vi "log analysis_gps.vi"() -> ()   [LabVIEW 2018] (continued)
2 27.900000 0 0\trobot status\t233.917361\t102.956881\t8.394900\t0.257932\t-0.250093\t-19.886143\t0.214000\t0.155000\n\t\n15:20:07.4\tlog_raw\tgps_raw\t\tsystem status\tnormal 2 27.900000 0 0\trobot status\t234.044213\t102.902455\t8.392800\t0.335822\t-0.062478\t-19.109713\t0.317000\t-0.011000\n\t\n15:20:07.9\tlog_raw\tgps_raw\t\tsystem status\tnormal 2 27.900000 0 0\trobot status\t234.173574\t102.852025\t8.391200\t0.185875\t0.011121\t-18.240384\t0.261000\t0.072000\n\t\n15:20:08.4\tlog_raw\tgps_raw\t\tsystem status\tnormal 2 27.900000 0 0\trobot status\t234.306855\t102.799992\t8.389600\t0.221268\t0.001420\t-17.502201\t0.351000\t-0.068000\n\t\n15:20:08.9\tlog_raw\tgps_raw\t#INSPVAXA,USB3,0,49.0,FINESTEERING,2107,282026.900,02000000,471d,15824;INS_ALIGNMENT_COMPLETE,INS_RTKFIXED,37.37105597447,126.72348196925,8.3886,22.3000,-0.1101,0.2823,-0.0032,0.311492548,-0.004113518,106.939400218,0.4050,0.2960,0.5269,0.1087,0.0927,0.0760,0.1504,0.1513,4.9517,0f000001,0*e3da5464\n\tsystem status\tnormal 2 27.900000 0 0\trobot status\t234.454891\t102.743810\t8.388600\t0.311493\t-0.004114\t-16.939400\t0.243000\t0.103000\n\t\n15:20:09.4\tlog_raw\tgps_raw\t\tsystem status\tnormal 2 27.900000 0 0\trobot status\t234.572623\t102.698923\t8.387800\t0.503029\t-0.025580\t-16.641655\t0.366000\t-0.093000\n\t\n15:20:09.9\tlog_raw\tgps_raw\t\tsystem status\tnormal 2 28.000000 0 0\trobot status\t234.705268\t102.650315\t8.386900\t0.470119\t-0.136101\t-16.414605\t0.222000\t0.114000\n\t\n15:20:10.4\tlog_raw\tgps_raw\t\tsystem status\tnormal 2 28.000000 0 0\trobot status\t234.841052\t102.602660\t8.385400\t0.352834\t-0.219751\t-16.257896\t0.249000\t0.066000\n\t\n15:20:10.9\tlog_raw\tgps_raw\t#INSPVAXA,USB3,0,48.5,FINESTEERING,2107,282028.900,02000000,471d,15824;INS_ALIGNMENT_COMPLETE,INS_RTKFIXED,37.37105423586,126.72348799189,8.3853,22.3000,-0.0954,0.2609,0.0063,0.345591384,-0.136100185,106.270510244,0.4039,0.2954,0.5254,0.1083,0.0924,0.0759,0.1502,0.1513,4.9544,0f000001,0*0554cafd\n\tsystem status\tnormal 2 28.100000 0 0\trobot status\t234.988367\t102.550836\t8.385300\t0.345591\t-0.136100\t-16.270510\t0.353000\t-0.085000\n\t\n15:20:11.4\tlog_raw\tgps_raw\t#INSPVAXA,USB3,0,51.5,FINESTEERING,2107,282029.400,02000000,471d,15824;INS_ALIGNMENT_COMPLETE,INS_RTKFIXED,37.37105381452,126.72348943964,8.3855,22.3000,-0.0956,0.2580,0.0057,0.437004372,-0.047146220,106.316911709,0.4029,0.2951,0.5243,0.1082,0.0924,0.0758,0.1501,0.1513,4.9556,0f000001,0*8a2f1e39\n\tsystem status\tnormal 2 28.100000 0 0\trobot status\t235.116606\t102.504071\t8.385500\t0.437004\t-0.047146\t-16.316912\t0.290000\t-0.013000\n\t\n15:20:11.9\tlog_raw\tgps_raw\t\tsystem status\tnormal 2 28.100000 0 0\trobot status\t235.235324\t102.460737\t8.385200\t0.512593\t-0.025982\t-16.425226\t0.294000\t-0.033000\n\t\n15:20:12.4\tlog_raw\tgps_raw\t\tsystem status\tnormal 2 28.100000 0 0\trobot status\t235.364702\t102.414096\t8.385200\t0.428006\t0.220406\t-16.561656\t0.296000\t-0.023000\n\t\n15:20:12.9\tlog_raw\tgps_raw\t\tsystem status\tnormal 2 28.100000 0 0\trobot status\t235.492637\t102.367047\t8.386000\t0.390693\t0.448694\t-16.706600\t0.298000\t-0.026000\n\t\n15:20:13.4\tlog_raw\tgps_raw\t\tsystem status\tnormal 2 28.100000 0 0\trobot status\t235.625886\t102.316793\t8.387700\t0.367788\t0.548182\t-16.923819\t0.298000\t-0.028000\n\t\n15:20:13.9\tlog_raw\tgps_raw\t\tsystem status\tnormal 2 28.100000 0 0\trobot status\t235.772529\t102.261880\t8.389500\t0.368907\t0.593009\t-17.130750\t0.304000\t-0.029000\n\t\n15:20:14.4\tlog_raw\tgps_raw\t#INSPVAXA,USB3,0,49.5,FINESTEERING,2107,282032.400,02000000,471d,15824;INS_ALIGNMENT_COMPLETE,INS_RTKFIXED,37.37105111138,126.72349854734,8.3925,22.3000,-0.1007,0.2882,0.0025,0.307227666,0.473154463,107.541908960,0.4011,0.2941,0.5198,0.1079,0.0924,0.0756,0.1501,0.1513,4.9577,0f000001,0*dbe53f25\n\tsystem status\tnormal 2 28.100000 0 0\trobot status\t235.923351\t102.204041\t8.392500\t0.307228\t0.473154\t-17.541909\t0.297000\t-0.033000\n\t\n15:20:14.9\tlog_raw\tgps_raw\t\tsystem status\tnormal 2 28.100000 0 0\trobot status\t236.048053\t102.155485\t8.396300\t0.259641\t0.471756\t-17.852264\t0.249000\t-0.099000\n\t\n15:20:15.4\tlog_raw\tgps_raw\t#INSPVAXA,USB3,0,50.0,FINESTEERING,2107,282033.400,02008000,471d,15824;INS_ALIGNMENT_COMPLETE,INS_RTKFIXED,37.37105012658,126.72350166762,8.4012,22.3000,-0.1057,0.2825,0.0064,0.046728519,0.492534824,108.559226244,0.4006,0.2938,0.5182,0.1078,0.0924,0.0755,0.1501,0.1512,4.9578,0f000001,0*3bd3df90\n\tsystem status\tnormal 2 28.000000 0 0\trobot status\t236.199741\t102.094735\t8.401200\t0.046729\t0.492535\t-18.559226\t0.359000\t0.057000\n\t\n15:20:15.9\tlog_raw\tgps_raw\t#INSPVAXA,USB3,0,50.0,FINESTEERING,2107,282033.900,02008000,471d,15824;INS_ALIGNMENT_COMPLETE,INS_RTKFIXED,37.37104960391,126.72350321994,8.4050,22.3000,-0.1156,0.2745,0.0097,0.015907780,0.376843772,109.332052646,0.4006,0.2938,0.5182,0.1078,0.0924,0.0755,0.1501,0.1512,4.9578,0f000001,0*2158b20c\n\tsystem status\tnormal 2 28.000000 0 0\trobot status\t236.337243\t102.036723\t8.405000\t0.015908\t0.376844\t-19.332053\t0.278000\t-0.059000\n\t\n15:20:16.4\tlog_raw\tgps_raw\t#INSPVAXA,USB3,0,47.5,FINESTEERING,2107,282034.400,02008000,471d,15824;INS_ALIGNMENT_COMPLETE,INS_RTKFIXED,37.37104906846,126.72350474212,8.4070,22.3000,-0.1192,0.2804,0.0105,-0.067520061,0.436867001,110.176313539,0.4000,0.2937,0.5167,0.1078,0.0924,0.0754,0.1502,0.1512,4.9578,0f000001,0*936b6da1\n\tsystem status\tnormal 2 28.000000 0 0\trobot status\t236.472075\t101.977293\t8.407000\t-0.067520\t0.436867\t-20.176314\t0.309000\t-0.023000\n\t\n15:20:16.9\tlog_raw\tgps_raw\t\tsystem status\tnormal 2 27.900000 0 0\trobot status\t236.591378\t101.923007\t8.409200\t-0.152287\t0.519773\t-20.980713\t0.257000\t-0.095000\n\t\n15:20:17.4\tlog_raw\tgps_raw\t#INSPVAXA,USB3,0,48.0,FINESTEERING,2107,282035.400,02008000,471d,15824;INS_ALIGNMENT_COMPLETE,INS_RTKFIXED,37.37104794270,126.72350775630,8.4115,22.3000,-0.1276,0.2808,0.0020,-0.201006751,0.469956354,111.990081929,0.3992,0.2935,0.5154,0.1077,0.0923,0.0754,0.1502,0.1511,4.9577,0f000001,0*ad6b63a0\n\tsystem status\tnormal 2 27.900000 0 0\trobot status\t236.739066\t101.852343\t8.411500\t-0.201007\t0.469956\t-21.990082\t0.317000\t-0.026000\n\t\n15:20:17.9\tlog_raw\tgps_raw\t#INSPVAXA,USB3,0,48.0,FINESTEERING,2107,282035.900,02008000,471d,15824;INS_ALIGNMENT_COMPLETE,INS_RTKFIXED,37.37104734832,126.72350923933,8.4125,22.3000,-0.1168,0.2783,-0.0124,-0.218567372,0.308742852,112.764094273,0.3992,0.2935,0.5154,0.1077,0.0923,0.0754,0.1502,0.1511,4.9577,0f000001,0*3d3cbf81\n\tsystem status\tnormal 2 28.000000 0 0\trobot status\t236.870430\t101.786372\t8.412500\t-0.218567\t0.308743\t-22.764094\t0.245000\t-0.119000\n\t\n15:20:18.4\tlog_raw\tgps_raw\t\tsystem status\tnormal 2 28.000000 0 0\trobot status\t236.986821\t101.725685\t8.413100\t-0.337267\t0.288547\t-23.353363\t0.373000\t0.077000\n\t\n15:20:18.9\tlog_raw\tgps_raw\t#INSPVAXA,USB3,0,50.0,FINESTEERING,2107,282036.900,02008000,471d,15824;INS_ALIGNMENT_COMPLETE,INS_RTKFIXED,37.37104611251,126.72351217399,8.4148,22.3000,-0.1294,0.2583,0.0040,-0.390769339,0.147574689,113.900095191,0.3984,0.2933,0.5139,0.1077,0.0919,0.0753,0.1502,0.1511,4.9576,0f000001,0*94857a61\n\tsystem status\tnormal 2 28.000000 0 0\trobot status\t237.130378\t101.649209\t8.414800\t-0.390769\t0.147575\t-23.900095\t0.341000\t0.060000\n\t\n15:20:19.4\tlog_raw\tgps_raw\t#INSPVAXA,USB3,0,48.0,FINESTEERING,2107,282037.400,02000000,471d,15824;INS_ALIGNMENT_COMPLETE,INS_RTKFIXED,37.37104547793,126.72351361006,8.4177,22.3000,-0.1348,0.2688,0.0058,-0.392403190,0.136695016,114.188183924,0.3974,0.2930,0.5127,0.1077,0.0918,0.0752,0.1502,0.1510,4.9580,0f000001,0*b3a6b226\n\tsystem status\tnormal 2 28.000000 0 0\trobot status\t237.257582\t101.578777\t8.417700\t-0.392403\t0.136695\t-24.188184\t0.293000\t-0.014000\n\t\n15:20:19.9\tlog_raw\tgps_raw\t#INSPVAXA,USB3,0,48.0,FINESTEERING,2107,282037.900,02000000,471d,15824;INS_ALIGNMENT_COMPLETE,INS_RTKFIXED,37.37104482885,126.72351504265,8.4195,22.3000,-0.1327,0.2535,0.0065,-0.334026852,0.167702494,114.415099877,0.3974,0.2930,0.5127,0.1077,0.0918,0.0752,0.1502,0.1510,4.9580,0f000001,0*e3ab242e\n\tsystem status\tnormal 2 28.100000 0 0\trobot status\t237.384479\t101.506735\t8.419500\t-0.334027\t0.167702\t-24.415100\t0.276000\t-0.018000\n\t\n15:20:20.4\tlog_raw\tgps_raw\t#INSPVAXA,USB3,0,48.5,FINESTEERING,2107,282038.400,02000000,471d,15824;INS_ALIGNMENT_COMPLETE,INS_RTKFIXED,37.37104419976,126.72351643213,8.4201,22.3000,-0.1292,0.2573,0.0088,-0.447214076,0.203710277,114.641680201,0.3969,0.2929,0.5120,0.1077,0.0919,0.0752,0.1502,0.1510,4.9585,0f000001,0*5ffb5d5a\n\tsystem status\tnormal 2 28.100000 0 0\trobot status\t237.507557\t101.436913\t8.420100\t-0.447214\t0.203710\t-24.641680\t0.295000\t0.006000\n\t\n15:20:20.9\tlog_raw\tgps_raw\t#INSPVAXA,USB3,0,48.5,FINESTEERING,2107,282038.900,02000000,471d,15824;INS_ALIGNMENT_COMPLETE,INS_RTKFIXED,37.37104355987,126.72351779908,8.4210,22.3000,-0.1397,0.2477,0.0110,-0.380183542,0.075701801,114.791210844,0.3969,0.2929,0.5120,0.1077,0.0919,0.0752,0.1502,0.1510,4.9585,0f000001,0*4f3052be\n\tsystem status\tnormal 2 28.100000 0 0\trobot status\t237.628639\t101.365891\t8.421000\t-0.380184\t0.075702\t-24.791211\t0.298000\t0.012000\n\t\n15:20:21.4\tlog_raw\tgps_raw\t#INSPVAXA,USB3,0,49.5,FINESTEERING,2107,282039.400,02000000,471d,15824;INS_ALIGNMENT_COMPLETE,INS_RTKFIXED,37.37104291933,126.72351914927,8.4230,22.3000,-0.1461,0.2586,0.0054,-0.203449941,0.032639383,114.880489837,0.3965,0.2928,0.5114,0.1077,0.0919,0.0752,0.1501,0.1510,4.9590,0f000001,0*7f207efe\n\tsystem status\tnormal 2 28.100000 0 0\trobot status\t237.748237\t101.294798\t8.423000\t-0.203450\t0.032639\t-24.880490\t0.302000\t0.021000\n\t\n15:20:21.9\tlog_raw\tgps_raw\t#INSPVAXA,USB3,0,49.5,FINESTEERING,2107,282039.900,02000000,471d,15824;INS_ALIGNMENT_COMPLETE,INS_RTKFIXED,37.37104224465,126.72352058384,8.4263,22.3000,-0.1547,0.2700,0.0148,-0.050110889,-0.053478733,114.971719756,0.3965,0.2928,0.5114,0.1077,0.0919,0.0752,0.1501,0.1510,4.9590,0f000001,0*a22ed322\n\tsystem status\tnormal 2 28.100000 0 0\trobot status\t237.875308\t101.219915\t8.426300\t-0.050111\t-0.053479\t-24.971720\t0.298000\t0.021000\n\t\n15:20:22.4\tlog_raw\tgps_raw\t#INSPVAXA,USB3,0,45.0,FINESTEERING,2107,282040.400,02000000,471d,15824;INS_ALIGNMENT_COMPLETE,INS_RTKFIXED,37.37104154925,126.72352205735,8.4266,22.3000,-0.1535,0.2759,0.0134,0.069839878,-0.109167571,115.012196802,0.3963,0.2927,0.5107,0.1078,0.0920,0.0752,0.1500,0.1510,4.9596,0f000001,0*a12699f2\n\tsystem status\tnormal 2 28.100000 0 0\trobot status\t238.005830\t101.142733\t8.426600\t0.069840\t-0.109168\t-25.012197\t0.313000\t0.006000\n\t\n15:20:22.9\tlog_raw\tgps_raw\t#INSPVAXA,USB3,0,45.0,FINESTEERING,2107,282040.900,02000000,471d,15824;INS_ALIGNMENT_COMPLETE,INS_RTKFIXED,37.37104084785,126.72352353291,8.4256,22.3000,-0.1448,0.2740,0.0009,0.161796846,-0.076999668,115.007657548,0.3963,0.2927,0.5107,0.1078,0.0920,0.0752,0.1500,0.1510,4.9596,0f000001,0*3a67e90b\n\tsystem status\tnormal 2 28.100000 0 0\trobot status\t238.136532\t101.064884\t8.425600\t0.161797\t-0.077000\t-25.007658\t0.302000\t0.043000\n\t\n15:20:23.4\tlog_raw\tgps_raw\t#INSPVAXA,USB3,0,50.0,FINESTEERING,2107,282041.400,02000000,471d,15824;INS_ALIGNMENT_COMPLETE,INS_RTKFIXED,37.37104019644,126.72352491689,8.4246,22.3000,-0.1518,0.2723,-0.0022,0.212334944,-0.070041433,114.640487697,0.3961,0.2927,0.5104,0.1077,0.0921,0.0751,0.1499,0.1510,4.9600,0f000001,0*8b513f40\n\tsystem status\tnormal 2 28.000000 0 0\trobot status\t238.259123\t100.992584\t8.424600\t0.212335\t-0.070041\t-24.640488\t0.375000\t-0.076000\n\t\n15:20:23.9\tlog_raw\tgps_raw\t#INSPVAXA,USB3,0,50.0,FINESTEERING,2107,282041.900,02000000,471d,15824;INS_ALIGNMENT_COMPLETE,INS_RTKFIXED,37.37103955120,126.72352632757,8.4231,22.3000,-0.1599,0.2675,-0.0000,0.251612681,-0.024570483,114.066468030,0.3961,0.2927,0.5104,0.1077,0.0921,0.0751,0.1499,0.1510,4.9600,0f000001,0*ee21d353\n\tsystem status\tnormal 2 27.900000 0 0\trobot status\t238.384079\t100.920969\t8.423100\t0.251613\t-0.024570\t-24.066468\t0.317000\t0.005000\n\t\n15:20:24.4\tlog_raw\tgps_raw\t\tsystem status\tnormal 2 27.800000 0 0\trobot status\t238.495736\t100.858105\t8.423100\t0.406731\t0.010002\t-23.314874\t0.448000\t-0.179000\n\t\n15:20:24.9\tlog_raw\tgps_raw\t\tsystem status\tnormal 2 27.800000 0 0\trobot status\t238.616533\t100.791763\t8.422800\t0.572531\t0.213158\t-22.278108\t0.294000\t0.064000\n\t\n15:20:25.4\tlog_raw\tgps_raw\t#INSPVAXA,USB3,0,49.0,FINESTEERING,2107,282043.400,02000000,471d,15824;INS_ALIGNMENT_COMPLETE,INS_RTKFIXED,37.37103775397,126.72353053671,8.4224,22.3000,-0.1356,0.2719,-0.0039,0.469507443,0.217168676,111.114657761,0.4278,0.2934,0.5225,0.1125,0.0922,0.0761,0.1498,0.1516,4.9609,0f000001,0*26bfa601\n\tsystem status\tnormal 2 27.800000 0 0\trobot status\t238.756917\t100.721493\t8.422400\t0.469507\t0.217169\t-21.114658\t0.292000\t0.049000\n\t\n15:20:25.9\tlog_raw\tgps_raw\t#INSPVAXA,USB3,0,49.0,FINESTEERING,2107,282043.900,02000000,471d,15824;INS_ALIGNMENT_COMPLETE,INS_RTKFIXED,37.37103719773,126.72353199656,8.4232,22.3000,-0.1151,0.2555,0.0099,0.378672959,0.355237505,110.161764009,0.4278,0.2934,0.5225,0.1125,0.0922,0.0761,0.1498,0.1516,4.9609,0f000001,0*a56cfb0a\n\tsystem status\tnormal 2 27.800000 0 0\trobot status\t238.886228\t100.659756\t8.423200\t0.378673\t0.355238\t-20.161764\t0.371000\t-0.074000\n\t\n15:20:26.4\tlog_raw\tgps_raw\t#INSPVAXA,USB3,0,49.0,FINESTEERING,2107,282044.400,02000000,471d,15824;INS_ALIGNMENT_COMPLETE,INS_RTKFIXED,37.37103668630,126.72353343626,8.4255,22.3000,-0.1146,0.2521,0.0005,0.230484735,0.495195972,109.291973317,0.4151,0.2930,0.5192,0.1093,0.0918,0.0756,0.1496,0.1511,4.9617,0f000001,0*69c2d113\n\tsystem status\tnormal 2 27.800000 0 0\trobot status\t239.013755\t100.602991\t8.425500\t0.230485\t0.495196\t-19.291973\t0.232000\t0.135000\n\t\n15:20:26.9\tlog_raw\tgps_raw\t#INSPVAXA,USB3,0,49.0,FINESTEERING,2107,282044.900,02000000,471d,15824;INS_ALIGNMENT_COMPLETE,INS_RTKFIXED,37.37103618153,126.72353489391,8.4287,22.3000,-0.1231,0.2600,0.0038,0.173840708,0.566394531,108.664354090,0.4151,0.2930,0.5192,0.1093,0.0918,0.0756,0.1496,0.1511,4.9617,0f000001,0*5975ddd2\n\tsystem status\tnormal 2 27.900000 0 0\trobot status\t239.142871\t100.546966\t8.428700\t0.173841\t0.566395\t-18.664354\t0.271000\t0.056000\n\t\n15:20:27.4\tlog_raw\tgps_raw\t#INSPVAXA,USB3,0,50.5,FINESTEERING,2107,282045.400,02000000,471d,15824;INS_ALIGNMENT_COMPLETE,INS_RTKFIXED,37.37103569365,126.72353637102,8.4304,22.3000,-0.1241,0.2677,0.0051,0.029985100,0.713380187,108.316777088,0.4073,0.2928,0.5168,0.1078,0.0917,0.0754,0.1495,0.1510,4.9629,0f000001,0*ed89f5e7\n\tsystem status\tnormal 2 27.900000 0 0\trobot status\t239.273711\t100.492815\t8.430400\t0.029985\t0.713380\t-18.316777\t0.224000\t0.108000\n\t\n15:20:27.9\tlog_raw\tgps_raw\t#INSPVAXA,USB3,0,50.5,FINESTEERING,2107,282045.900,02000000,471d,15824;INS_ALIGNMENT_COMPLETE,INS_RTKFIXED,37.37103520329,126.72353786687,8.4303,22.3000,-0.1276,0.2596,0.0072,-0.128043744,0.852574922,108.131029460,0.4073,0.2928,0.5168,0.1078,0.0917,0.0754,0.1495,0.1510,4.9629,0f000001,0*d9490397\n\tsystem status\tnormal 2 28.000000 0 0\trobot status\t239.406211\t100.438389\t8.430300\t-0.128044\t0.852575\t-18.131029\t0.243000\t0.073000\n\t\n15:20:28.4\tlog_raw\tgps_raw\t#INSPVAXA,USB3,0,47.5,FINESTEERING,2107,282046.400,02000000,471d,15824;INS_ALIGNMENT_COMPLETE,INS_RTKFIXED,37.37103472430,126.72353933486,8.4326,22.3000,-0.1274,0.2469,0.0233,-0.197512090,0.856787490,108.035575182,0.4031,0.2927,0.5152,0.1074,0.0918,0.0753,0.1494,0.1509,4.9644,0f000001,0*7594b79a\n\tsystem status\tnormal 2 28.100000 0 0\trobot status\t239.536243\t100.385224\t8.432600\t-0.197512\t0.856787\t-18.035575\t0.267000\t0.040000\n\t\n15:20:28.9\tlog_raw\tgps_raw\t#INSPVAXA,USB3,0,47.5,FINESTEERING,2107,282046.900,02000000,471d,15824;INS_ALIGNMENT_COMPLETE,INS_RTKFIXED,37.37103423045,126.72354082894,8.4356,22.3000,-0.1317,0.2525,0.0181,-0.272615220,0.680276177,108.135899637,0.4031,0.2927,0.5152,0.1074,0.0918,0.0753,0.1494,0.1509,4.9644,0f000001,0*0ad6ca19\n\tsystem status\tnormal 2 28.100000 0 0\trobot status\t239.668586\t100.330411\t8.435600\t-0.272615\t0.680276\t-18.135900\t0.287000\t-0.001000\n\t\n15:20:29.4\tlog_raw\tgps_raw\t#INSPVAXA,USB3,0,50.0,FINESTEERING,2107,282047.400,02000000,471d,15824;INS_ALIGNMENT_COMPLETE,INS_RTKFIXED,37.37103373575,126.72354228047,8.4378,22.3000,-0.1209,0.2496,0.0116,-0.304500119,0.597497624,108.265546221,0.4007,0.2928,0.5142,0.1074,0.0918,0.0752,0.1494,0.1510,4.9658,0f000001,0*f7570865\n\tsystem status\tnormal 2 28.100000 0 0\trobot status\t239.797160\t100.275503\t8.437800\t-0.304500\t0.597498\t-18.265546\t0.300000\t-0.019000\n\t\n15:20:29.9\tlog_raw\tgps_raw\t#INSPVAXA,USB3,0,50.0,FINESTEERING,2107,282047.900,02000000,471d,15824;INS_ALIGNMENT_COMPLETE,INS_RTKFIXED,37.37103324070,126.72354372631,8.4396,22.3000,-0.1245,0.2634,0.0029,-0.432470862,0.435465093,108.449839156,0.4007,0.2928,0.5142,0.1074,0.0918,0.0752,0.1494,0.1510,4.9658,0f000001,0*36db7439\n\tsystem status\tnormal 2 28.100000 0 0\trobot status\t239.925231\t100.220557\t8.439600\t-0.432471\t0.435465\t-18.449839\t0.300000\t-0.018000\n\t\n15:20:30.4\tlog_raw\tgps_raw\t#INSPVAXA,USB3,0,50.5,FINESTEERING,2107,282048.400,02000000,471d,15824;INS_ALIGNMENT_COMPLETE,INS_RTKFIXED,37.37103276390,126.72354512195,8.4422,22.3000,-0.1174,0.2527,0.0035,-0.579219064,0.548453263,108.588640946,0.3999,0.2929,0.5136,0.1077,0.0919,0.0752,0.1494,0.1510,4.9669,0f000001,0*39dcb86d\n\tsystem status\tnormal 2 28.100000 0 0\trobot status\t240.048854\t100.167636\t8.442200\t-0.579219\t0.548453\t-18.588641\t0.300000\t-0.029000\n\t\n15:20:30.9\tlog_raw\tgps_raw\t#INSPVAXA,USB3,0,50.5,FINESTEERING,2107,282048.900,02000000,471d,15824;INS_ALIGNMENT_COMPLETE,INS_RTKFIXED,37.37103224560,126.72354663214,8.4444,22.3000,-0.1277,0.2757,0.0017,-0.626592157,0.566170063,108.836719215,0.3999,0.2929,0.5136,0.1077,0.0919,0.0752,0.1494,0.1510,4.9669,0f000001,0*2908ea23\n\tsystem status\tnormal 2 28.100000 0 0\trobot status\t240.182624\t100.110108\t8.444400\t-0.626592\t0.566170\t-18.836719\t0.298000\t-0.029000\n\t\n15:20:31.4\tlog_raw\tgps_raw\t#INSPVAXA,USB3,0,49.5,FINESTEERING,2107,282049.400,02000000,471d,15824;INS_ALIGNMENT_COMPLETE,INS_RTKFIXED,37.37103169688,126.72354817389,8.4462,22.3000,-0.1370,0.2620,0.0032,-0.416455659,0.615214543,109.052473427,0.3987,0.2929,0.5129,0.1079,0.0918,0.0751,0.1495,0.1510,4.9681,0f000001,0*9e3ef17b\n\tsystem status\tnormal 2 28.100000 0 0\trobot status\t240.319190\t100.049205\t8.446200\t-0.416456\t0.615215\t-19.052473\t0.297000\t-0.023000\n\t\n15:20:31.9\tlog_raw\tgps_raw\t#INSPVAXA,USB3,0,49.5,FINESTEERING,2107,282049.900,02000000,471d,15824;INS_ALIGNMENT_COMPLETE,INS_RTKFIXED,37.37103115870,126.72354965807,8.4484,22.3000,-0.1429,0.2729,-0.0002,-0.328473070,0.641311301,109.380425466,0.3987,0.2929,0.5129,0.1079,0.0918,0.0751,0.1495,0.1510,4.9681,0f000001,0*d7629724\n\tsystem status\tnormal 2 28.100000 0 0\trobot status\t240.450656\t99.989471\t8.448400\t-0.328473\t0.641311\t-19.380425\t0.309000\t-0.016000\n\t\n15:20:32.4\tlog_raw\tgps_raw\t#INSPVAXA,USB3,0,50.0,FINESTEERING,2107,282050.400,02000000,471d,15824;INS_ALIGNMENT_COMPLETE,INS_RTKFIXED,37.37103062705,126.72355118407,8.4512,22.3000,-0.1472,0.2693,0.0005,-0.421432718,0.551827258,109.755848199,0.3977,0.2928,0.5121,0.1079,0.0919,0.0751,0.1495,0.1509,4.9692,0f000001,0*9b0507cc\n\tsystem status\tnormal 2 28.100000 0 0\trobot status\t240.585827\t99.930463\t8.451200\t-0.421433\t0.551827\t-19.755848\t0.285000\t-0.038000\n\t\n15:20:32.9\tlog_raw\tgps_raw\t#INSPVAXA,USB3,0,50.0,FINESTEERING,2107,282050.900,02000000,471d,15824;INS_ALIGNMENT_COMPLETE,INS_RTKFIXED,37.37103009197,126.72355271256,8.4539,22.3000,-0.1417,0.2757,0.0094,-0.635318550,0.518176153,110.294243776,0.3977,0.2928,0.5121,0.1079,0.0919,0.0751,0.1495,0.1509,4.9692,0f000001,0*281a41b6\n\tsystem status\tnormal 2 28.000000 0 0\trobot status\t240.721218\t99.871073\t8.453900\t-0.635319\t0.518176\t-20.294244\t0.313000\t-0.005000\n\t\n15:20:33.4\tlog_raw\tgps_raw\t#INSPVAXA,USB3,0,48.0,FINESTEERING,2107,282051.400,02000000,471d,15824;INS_ALIGNMENT_COMPLETE,INS_RTKFIXED,37.37102952977,126.72355418303,8.4573,22.3000,-0.1452,0.2608,-0.0009,-0.446409440,0.466780038,110.936496346,0.3976,0.2929,0.5117,0.1080,0.0918,0.0751,0.1495,0.1509,4.9703,0f000001,0*e106e6fe\n\tsystem status\tnormal 2 28.000000 0 0\trobot status\t240.851470\t99.808674\t8.457300\t-0.446409\t0.466780\t-20.936496\t0.283000\t-0.053000\n\t\n15:20:33.9\tlog_raw\tgps_raw\t#INSPVAXA,USB3,0,48.0,FINESTEERING,2107,282051.900,02000000,471d,15824;INS_ALIGNMENT_COMPLETE,INS_RTKFIXED,37.37102892561,126.72355566978,8.4607,22.3000,-0.1442,0.2601,0.0120,-0.193968959,0.359112496,111.726524346,0.3976,0.2929,0.5117,0.1080,0.0918,0.0751,0.1495,0.1509,4.9703,0f000001,0*bd701264\n\tsystem status\tnormal 2 27.900000 0 0\trobot status\t240.983164\t99.741618\t8.460700\t-0.193969\t0.359112\t-21.726524\t0.304000\t-0.030000\n\t\n15:20:34.4\tlog_raw\tgps_raw\t#INSPVAXA,USB3,0,46.5,FINESTEERING,2107,282052.400,02000000,471d,15824;INS_ALIGNMENT_COMPLETE,INS_RTKFIXED,37.37102834660,126.72355712345,8.4631,22.3000,-0.1344,0.2420,0.0090,-0.254926417,0.436150918,112.550580060,0.3973,0.2929,0.5110,0.1078,0.0918,0.0751,0.1495,0.1508,4.9714,0f000001,0*49726e9c\n\tsystem status\tnormal 2 27.900000 0 0\trobot status\t241.111927\t99.677353\t8.463100\t-0.254926\t0.436151\t-22.550580\t0.309000\t-0.019000\n\t\n15:20:34.9\tlog_raw\tgps_raw\t#INSPVAXA,USB3,0,46.5,FINESTEERING,2107,282052.900,02000000,471d,15824;INS_ALIGNMENT_COMPLETE,INS_RTKFIXED,37.37102775131,126.72355855890,8.4646,22.3000,-0.1511,0.2448,0.0254,-0.250642756,0.477147225,113.358906308,0.3973,0.2929,0.5110,0.1078,0.0918,0.0751,0.1495,0.1508,4.9714,0f000001,0*ce9979aa\n\tsystem status\tnormal 2 27.900000 0 0\trobot status\t241.239077\t99.611281\t8.464600\t-0.250643\t0.477147\t-23.358906\t0.218000\t-0.135000\n\t\n15:20:35.4\tlog_raw\tgps_raw\t#INSPVAXA,USB3,0,44.5,FINESTEERING,2107,282053.400,02000000,471d,15824;INS_ALIGNMENT_COMPLETE,INS_RTKFIXED,37.37102714809,126.72355999231,8.4667,22.3000,-0.1605,0.2545,0.0109,-0.233782899,0.571505620,114.141889462,0.3971,0.2928,0.5106,0.1077,0.0917,0.0750,0.1495,0.1507,4.9724,0f000001,0*6bed7872\n\tsystem status\tnormal 2 28.000000 0 0\trobot status\t241.366046\t99.544329\t8.466700\t-0.233783\t0.571506\t-24.141889\t0.260000\t-0.071000\n\t\n15:20:35.9\tlog_raw\tgps_raw\t#DUALANTENNAHEADINGA,USB3,0,44.5,FINESTEERING,2107,282053.900,02000000,d426,15824;SOL_COMPUTED,NARROW_FLOAT,-1.000000000,165.380935669,31.219970703,0.0,261.390197754,180.000000000,\"631T\",19,7,7,7,04,00,20,03*4f993fc4\n\tsystem status\tnormal 2 28.000000 0 0\trobot status\t241.491285\t99.475212\t8.469300\t-0.027449\t0.599510\t-24.756735\t0.392000\t0.115000\n\t\n15:20:36.4\tlog_raw\tgps_raw\t#INSPVAXA,USB3,0,48.0,FINESTEERING,2107,282054.400,02000000,471d,15824;INS_ALIGNMENT_COMPLETE,INS_RTKFIXED,37.37102588447,126.72356281881,8.4708,22.3000,-0.1681,0.2698,0.0199,0.211462800,0.565070170,115.259101386,0.3974,0.2928,0.5104,0.1076,0.0917,0.0751,0.1495,0.1506,4.9735,0f000001,0*fe4062de\n\tsystem status\tnormal 2 28.000000 0 0\trobot status\t241.616413\t99.404080\t8.470800\t0.211463\t0.565070\t-25.259101\t0.273000\t-0.056000\n\t\n15:20:36.9\tlog_raw\tgps_raw\t#INSPVAXA,USB3,0,48.0,FINESTEERING,2107,282054.900,02000000,471d,15824;INS_ALIGNMENT_COMPLETE,INS_RTKFIXED,37.37102524848,126.72356421796,8.4709,22.3000,-0.1622,0.2530,-0.0006,0.102305423,0.525752233,115.651365939,0.3974,0.2928,0.5104,0.1076,0.0917,0.0751,0.1495,0.1506,4.9735,0f000001,0*0e3012d6\n\tsystem status\tnormal 2 28.000000 0 0\trobot status\t241.740347\t99.333491\t8.470900\t0.102305\t0.525752\t-25.651366\t0.362000\t0.073000\n\t\n15:20:37.4\tlog_raw\tgps_raw\t#INSPVAXA,USB3,0,46.5,FINESTEERING,2107,282055.400,02000000,471d,15824;INS_ALIGNMENT_COMPLETE,INS_RTKFIXED,37.37102459483,126.72356562736,8.4700,22.3000,-0.1625,0.2569,-0.0075,0.070588481,0.412699361,115.906103651,0.4155,0.2932,0.5168,0.1107,0.0919,0.0756,0.1495,0.1510,4.9747,0f000001,0*738f8c7d\n\tsystem status\tnormal 2 28.100000 0 0\trobot status\t241.865190\t99.260942\t8.470000\t0.070588\t0.412699\t-25.906104\t0.276000\t-0.031000\n\t\n15:20:37.9\tlog_raw\tgps_raw\t#INSPVAXA,USB3,0,46.5,FINESTEERING,2107,282055.900,02000000,471d,15824;INS_ALIGNMENT_COMPLETE,INS_RTKFIXED,37.37102394338,126.72356697461,8.4688,22.3000,-0.1600,0.2462,-0.0061,0.217668333,0.474174872,116.134195625,0.4155,0.2932,0.5168,0.1107,0.0919,0.0756,0.1495,0.1510,4.9747,0f000001,0*22c3b36b\n\tsystem status\tnormal 2 28.100000 0 0\trobot status\t241.984527\t99.188638\t8.468800\t0.217668\t0.474175\t-26.134196\t0.289000\t-0.006000\n\t\n15:20:38.4\tlog_raw\tgps_raw\t#INSPVAXA,USB3,0,48.0,FINESTEERING,2107,282056.400,02000000,471d,15824;INS_ALIGNMENT_COMPLETE,INS_RTKFIXED,37.37102326974,126.72356835081,8.4675,22.3000,-0.1698,0.2576,-0.0043,0.387693340,0.353581686,116.290488152,0.4308,0.2936,0.5243,0.1128,0.0921,0.0761,0.1495,0.1513,4.9761,0f000001,0*4bf67f5e\n\tsystem status\tnormal 2 28.100000 0 0\trobot status\t242.106428\t99.113871\t8.467500\t0.387693\t0.353582\t-26.290488\t0.301000\t0.003000\n\t\n15:20:38.9\tlog_raw\tgps_raw\t#DUALANTENNAHEADINGA,USB3,0,48.0,FINESTEERING,2107,282056.900,02000000,d426,15824;SOL_COMPUTED,L1_FLOAT,-1.000000000,188.034057617,48.521991730,0.0,149.833007813,180.000000000,\"631T\",17,7,7,7,04,00,20,03*4a1bc78c\n\tsystem status\tnormal 2 28.100000 0 0\trobot status\t242.226110\t99.040198\t8.466200\t0.418207\t0.298162\t-26.450377\t0.299000\t0.012000\n\t\n15:20:39.4\tlog_raw\tgps_raw\t#INSPVAXA,USB3,0,49.5,FINESTEERING,2107,282057.400,02000000,471d,15824;INS_ALIGNMENT_COMPLETE,INS_RTKFIXED,37.37102198176,126.72357104397,8.4666,22.3000,-0.1730,0.2276,-0.0046,0.296246592,0.281453997,116.587848153,0.4169,0.2930,0.5203,0.1094,0.0919,0.0756,0.1494,0.1507,4.9775,0f000001,0*365c3542\n\tsystem status\tnormal 2 28.100000 0 0\trobot status\t242.344984\t98.970918\t8.466600\t0.296247\t0.281454\t-26.587848\t0.291000\t0.014000\n\t\n15:20:39.9\tlog_raw\tgps_raw\t#INSPVAXA,USB3,0,49.5,FINESTEERING,2107,282057.900,02000000,471d,15824;INS_ALIGNMENT_COMPLETE,INS_RTKFIXED,37.37102132674,126.72357243204,8.4681,22.3000,-0.1784,0.2359,-0.0022,0.276182941,0.305119300,116.637377638,0.4169,0.2930,0.5203,0.1094,0.0919,0.0756,0.1494,0.1507,4.9775,0f000001,0*2cc7c943\n\tsystem status\tnormal 2 28.100000 0 0\trobot status\t242.467937\t98.898217\t8.468100\t0.276183\t0.305119\t-26.637378\t0.297000\t0.012000\n\t\n15:20:40.4\tlog_raw\tgps_raw\t#INSPVAXA,USB3,0,46.0,FINESTEERING,2107,282058.400,02000000,471d,15824;INS_ALIGNMENT_COMPLETE,INS_RTKFIXED,37.37102064028,126.72357384993,8.4690,22.3000,-0.1826,0.2708,0.0015,0.277724893,0.355072296,116.706780756,0.4085,0.2927,0.5173,0.1080,0.0919,0.0753,0.1493,0.1505,4.9788,0f000001,0*091434dc\n\tsystem status\tnormal 2 28.100000 0 0\trobot status\t242.593531\t98.822027\t8.469000\t0.277725\t0.355072\t-26.706781\t0.301000\t0.017000\n\t\n15:20:40.9\tlog_raw\tgps_raw\t#DUALANTENNAHEADINGA,USB3,0,46.0,FINESTEERING,2107,282058.900,02000000,d426,15824;SOL_COMPUTED,NARROW_FLOAT,-1.000000000,155.425567627,41.921077728,0.0,360.000000000,180.000000000,\"631T\",17,7,7,7,04,00,20,03*1ade94fd\n\tsystem status\tnormal 2 28.100000 0 0\trobot status\t242.720491\t98.744551\t8.468400\t0.118888\t0.350749\t-26.806059\t0.300000\t0.008000\n\t\n15:20:41.4\tlog_raw\tgps_raw\t#DUALANTENNAHEADINGA,USB3,0,47.5,FINESTEERING,2107,282059.400,02000000,d426,15824;SOL_COMPUTED,NARROW_FLOAT,-1.000000000,183.622436523,40.173770905,0.0,305.777679443,180.000000000,\"631T\",17,7,7,7,04,00,20,03*be7303c1\n\tsystem status\tnormal 2 28.100000 0 0\trobot status\t242.848183\t98.667062\t8.468100\t0.084829\t0.379264\t-26.775522\t0.333000\t-0.026000\n\t\n15:20:41.9\tlog_raw\tgps_raw\t#DUALANTENNAHEADINGA,USB3,0,47.5,FINESTEERING,2107,282059.900,02000000,d426,15824;SOL_COMPUTED,NARROW_FLOAT,-1.000000000,183.595245361,41.079216003,0.0,306.083618164,180.000000000,\"631T\",17,7,7,7,04,00,20,02*56ca6491\n\tsystem status\tnormal 2 28.100000 0 0\trobot status\t242.974228\t98.588998\t8.467700\t0.118036\t0.168442\t-26.656145\t0.265000\t0.060000\n\t\n15:20:42.4\tlog_raw\tgps_raw\t#DUALANTENNAHEADINGA,USB3,0,50.5,FINESTEERING,2107,282060.400,02000000,d426,15824;SOL_COMPUTED,L1_FLOAT,-1.000000000,188.621459961,32.809661865,0.0,201.470733643,180.000000000,\"631T\",16,6,6,6,04,00,20,02*4c9b8a65\n\tsystem status\tnormal 2 28.000000 0 0\trobot status\t243.097414\t98.513903\t8.469900\t0.221777\t0.034063\t-26.324180\t0.308000\t0.006000\n\t\n15:20:42.9\tlog_raw\tgps_raw\t#DUALANTENNAHEADINGA,USB3,0,50.5,FINESTEERING,2107,282060.900,02000000,d426,15824;SOL_COMPUTED,L1_FLOAT,-1.000000000,188.468612671,32.503238678,0.0,203.530487061,180.000000000,\"631T\",16,6,6,6,04,00,20,02*a42a0267\n\tsystem status\tnormal 2 28.000000 0 0\trobot status\t243.222876\t98.438864\t8.472300\t0.173018\t0.121987\t-25.847936\t0.342000\t-0.024000\n\t\n15:20:43.4\tlog_raw\tgps_raw\t#INSPVAXA,USB3,0,52.0,FINESTEERING,2107,282061.400,02000000,471d,15824;INS_ALIGNMENT_COMPLETE,INS_RTKFIXED,37.37101652600,126.72358236543,8.4736,22.3000,-0.1613,0.2499,-0.0018,0.130104122,0.184346259,115.264963296,0.3994,0.2931,0.5137,0.1077,0.0920,0.0751,0.1491,0.1505,4.9829,0f000001,0*84f4c641\n\tsystem status\tnormal 2 27.900000 0 0\trobot status\t243.347820\t98.365383\t8.473600\t0.130104\t0.184346\t-25.264963\t0.235000\t0.132000\n\t\n15:20:43.9\tlog_raw\tgps_raw\t#INSPVAXA,USB3,0,52.0,FINESTEERING,2107,282061.900,02000000,471d,15824;INS_ALIGNMENT_COMPLETE,INS_RTKFIXED,37.37101586728,126.72358376934,8.4724,22.3000,-0.1591,0.2551,-0.0023,0.208355260,0.306813184,114.636507713,0.3994,0.2931,0.5137,0.1077,0.0920,0.0751,0.1491,0.1505,4.9829,0f000001,0*6df399da\n\tsystem status\tnormal 2 27.900000 0 0\trobot status\t243.472177\t98.292272\t8.472400\t0.208355\t0.306813\t-24.636508\t0.258000\t0.088000\n\t\n15:20:44.4\tlog_raw\tgps_raw\t#DUALANTENNAHEADINGA,USB3,0,49.0,FINESTEERING,2107,282062.400,02000000,d426,15824;SOL_COMPUTED,NARROW_FLOAT,-1.000000000,152.663146973,-31.160461426,0.0,360.000000000,180.000000000,\"631T\",16,6,6,6,04,00,20,03*79a87a98\n\tsystem status\tnormal 2 28.000000 0 0\trobot status\t243.597454\t98.220964\t8.468900\t0.405613\t0.127349\t-23.918619\t0.311000\t0.000000\n\t\n15:20:44.9\tlog_raw\tgps_raw\t#INSPVAXA,USB3,0,49.0,FINESTEERING,2107,282062.900,02000000,471d,15824;INS_ALIGNMENT_COMPLETE,INS_RTKFIXED,37.37101460250,126.72358663230,8.4657,22.3000,-0.1655,0.2464,-0.0060,0.173361139,0.049133885,113.278518772,0.3984,0.2930,0.5124,0.1078,0.0919,0.0750,0.1489,0.1506,4.9845,0f000001,0*56ff342f\n\tsystem status\tnormal 2 27.900000 0 0\trobot status\t243.725773\t98.151893\t8.465700\t0.173361\t0.049134\t-23.278519\t0.293000\t0.012000\n\t\n15:20:45.4\tlog_raw\tgps_raw\t#INSPVAXA,USB3,0,50.0,FINESTEERING,2107,282063.400,02000000,471d,15824;INS_ALIGNMENT_COMPLETE,INS_RTKFIXED,37.37101399789,126.72358807716,8.4654,22.3000,-0.1571,0.2332,0.0025,0.071973073,0.119158160,112.739398614,0.3982,0.2929,0.5114,0.1079,0.0918,0.0750,0.1488,0.1506,4.9861,0f000001,0*f4c7a0fa\n\tsystem status\tnormal 2 28.000000 0 0\trobot status\t243.853756\t98.084787\t8.465400\t0.071973\t0.119158\t-22.739399\t0.203000\t0.125000\n\t\n15:20:45.9\tlog_raw\tgps_raw\t#DUALANTENNAHEADINGA,USB3,0,50.0,FINESTEERING,2107,282063.900,02000000,d426,15824;SOL_COMPUTED,NARROW_FLOAT,-1.000000000,151.658050537,-47.108062744,0.0,360.000000000,180.000000000,\"631T\",15,6,6,6,04,00,20,03*1e02ddce\n\tsystem status\tnormal 2 28.000000 0 0\trobot status\t243.981694\t98.018006\t8.466000\t0.119989\t0.224485\t-22.326644\t0.334000\t-0.050000\n\t\n15:20:46.4\tlog_raw\tgps_raw\t#INSPVAXA,USB3,0,49.5,FINESTEERING,2107,282064.400,02008000,471d,15824;INS_ALIGNMENT_COMPLETE,INS_RTKFIXED,37.37101278897,126.72359100387,8.4654,22.3000,-0.1602,0.2656,-0.0115,0.293522321,0.241172864,111.956840334,0.3974,0.2927,0.5103,0.1078,0.0917,0.0750,0.1488,0.1506,4.9877,0f000001,0*fae7c97d\n\tsystem status\tnormal 2 28.000000 0 0\trobot status\t244.112999\t97.950608\t8.465400\t0.293522\t0.241173\t-21.956840\t0.303000\t-0.010000\n\t\n15:20:46.9\tlog_raw\tgps_raw\t#DUALANTENNAHEADINGA,USB3,0,49.5,FINESTEERING,2107,282064.900,02008000,d426,15824;SOL_COMPUTED,NARROW_FLOAT,-1.000000000,152.203399658,-59.519470215,0.0,360.000000000,180.000000000,\"631T\",18,7,7,6,04,00,20,03*8e7f9ac2\n\tsystem status\tnormal 2 28.000000 0 0\trobot status\t244.244240\t97.884657\t8.462900\t0.262813\t0.426438\t-21.710783\t0.271000\t0.029000\n\t\n15:20:47.4\tlog_raw\tgps_raw\t#DUALANTENNAHEADINGA,USB3,0,49.5,FINESTEERING,2107,282065.400,02008000,d426,15824;SOL_COMPUTED,NARROW_FLOAT,-1.000000000,122.017272949,78.944664001,0.0,360.000000000,167.907485962,\"631T\",17,7,7,7,04,00,20,03*05083127\n\tsystem status\tnormal 2 28.000000 0 0\trobot status\t244.376049\t97.822681\t8.463300\t0.024783\t0.398209\t-21.682412\t0.261000\t0.046000\n\t\n15:20:47.9\tlog_raw\tgps_raw\t#DUALANTENNAHEADINGA,USB3,0,49.5,FINESTEERING,2107,282065.900,02008000,d426,15824;SOL_COMPUTED,NARROW_FLOAT,-1.000000000,121.918090820,78.941169739,0.0,360.000000000,169.045944214,\"631T\",18,7,7,7,04,00,20,03*3f11d063\n\tsystem status\tnormal 2 28.100000 0 0\trobot status\t244.510013\t97.758407\t8.464300\t-0.025799\t0.199451\t-21.704948\t0.356000\t-0.090000\n\t\n15:20:48.4\tlog_raw\tgps_raw\t#DUALANTENNAHEADINGA,USB3,0,48.0,FINESTEERING,2107,282066.400,02008000,d426,15824;SOL_COMPUTED,NARROW_FLOAT,-1.000000000,150.971466064,30.315032959,0.0,360.000000000,180.000000000,\"631T\",21,7,7,7,04,00,20,03*10224658\n\tsystem status\tnormal 2 28.100000 0 0\trobot status\t244.640455\t97.694857\t8.463700\t-0.125148\t0.100666\t-21.757399\t0.291000\t-0.013000\n\t\n15:20:48.9\tlog_raw\tgps_raw\t#DUALANTENNAHEADINGA,USB3,0,48.0,FINESTEERING,2107,282066.900,02008000,d426,15824;SOL_COMPUTED,NARROW_FLOAT,-1.000000000,150.582351685,29.219997406,0.0,360.000000000,180.000000000,\"631T\",21,7,7,7,04,00,20,03*814dc40f\n\tsystem status\tnormal 2 28.100000 0 0\trobot status\t244.773006\t97.628836\t8.461500\t-0.148107\t0.053469\t-21.841972\t0.293000\t-0.016000\n\t\n15:20:49.4\tlog_raw\tgps_raw\t#DUALANTENNAHEADINGA,USB3,0,50.0,FINESTEERING,2107,282067.400,02008000,d426,15824;SOL_COMPUTED,NARROW_FLOAT,-1.000000000,145.294387817,24.460121155,0.0,360.000000000,180.000000000,\"631T\",20,7,7,7,04,00,20,03*8bfd9c96\n\tsystem status\tnormal 2 28.100000 0 0\trobot status\t244.900254\t97.566780\t8.460200\t-0.186624\t-0.041449\t-21.938346\t0.297000\t-0.024000\n\t\n15:20:49.9\tlog_raw\tgps_raw\t#DUALANTENNAHEADINGA,USB3,0,50.0,FINESTEERING,2107,282067.900,02008000,d426,15824;SOL_COMPUTED,NARROW_FLOAT,-1.000000000,143.647583008,28.839637756,0.0,360.000000000,180.000000000,\"631T\",18,7,7,7,04,00,20,03*4514f4b2\n\tsystem status\tnormal 2 28.100000 0 0\trobot status\t245.030996\t97.502498\t8.459500\t-0.151914\t-0.106240\t-22.057241\t0.303000\t-0.018000\n\t\n15:20:50.4\tlog_raw\tgps_raw\t#INSPVAXA,USB3,0,47.0,FINESTEERING,2107,282068.400,02000000,471d,15824;INS_ALIGNMENT_COMPLETE,INS_RTKFIXED,37.37100819818,126.72360279226,8.4607,22.3000,-0.1621,0.2796,-0.0079,-0.283387467,0.022264293,112.218267949,0.3978,0.2926,0.5089,0.1077,0.0918,0.0750,0.1487,0.1505,4.9920,0f000001,0*2b60bbde\n\tsystem status\tnormal 2 28.100000 0 0\trobot status\t245.157196\t97.441070\t8.460700\t-0.283387\t0.022264\t-22.218268\t0.297000\t-0.016000\n\t\n15:20:50.9\tlog_raw\tgps_raw\t#DUALANTENNAHEADINGA,USB3,0,47.0,FINESTEERING,2107,282068.900,02000000,d426,15824;SOL_COMPUTED,NARROW_FLOAT,-1.000000000,100.644241333,68.634323120,0.0,360.000000000,124.100311279,\"631T\",21,7,7,7,04,00,20,03*c3cc83cc\n\tsystem status\tnormal 2 28.100000 0 0\trobot status\t245.290917\t97.374773\t8.462100\t-0.232449\t0.007242\t-22.472998\t0.296000\t-0.023000\n\t\n15:20:51.4\tlog_raw\tgps_raw\t#DUALANTENNAHEADINGA,USB3,0,46.5,FINESTEERING,2107,282069.400,02000000,d426,15824;SOL_COMPUTED,NARROW_FLOAT,-1.000000000,62.887535095,72.941581726,0.0,329.144042969,92.146186829,\"631T\",20,7,7,7,04,00,20,03*4ebf539f\n\tsystem status\tnormal 2 28.100000 0 0\trobot status\t245.424133\t97.309987\t8.463500\t-0.222890\t0.199740\t-22.702444\t0.302000\t-0.030000\n\t\n15:20:51.9\tlog_raw\tgps_raw\t#DUALANTENNAHEADINGA,USB3,0,46.5,FINESTEERING,2107,282069.900,02000000,d426,15824;SOL_COMPUTED,NARROW_FLOAT,-1.000000000,62.622955322,73.006401062,0.0,328.499725342,92.030387878,\"631T\",20,7,7,7,04,00,20,03*db3abc9d\n\tsystem status\tnormal 2 28.100000 0 0\trobot status\t245.556332\t97.245214\t8.465800\t-0.232901\t0.563527\t-22.885397\t0.296000\t-0.023000\n\t\n15:20:52.4\tlog_raw\tgps_raw\t#DUALANTENNAHEADINGA,USB3,0,42.0,FINESTEERING,2107,282070.400,02008000,d426,15824;SOL_COMPUTED,NARROW_FLOAT,-1.000000000,164.998916626,60.444377899,0.0,329.796081543,180.000000000,\"631T\",21,7,7,7,04,00,20,03*8640d9ed\n\tsystem status\tnormal 2 28.100000 0 0\trobot status\t245.687215\t97.178526\t8.468000\t-0.064960\t0.784682\t-23.158289\t0.310000\t-0.010000\n\t\n15:20:52.9\tlog_raw\tgps_raw\t#DUALANTENNAHEADINGA,USB3,0,42.0,FINESTEERING,2107,282070.900,02008000,d426,15824;SOL_COMPUTED,NARROW_FLOAT,-1.000000000,166.059432983,59.466281891,0.0,316.536041260,180.000000000,\"631T\",22,7,7,7,04,00,20,03*a557aca2\n\tsystem status\tnormal 2 28.100000 0 0\trobot status\t245.815046\t97.111177\t8.471300\t0.198069\t0.918051\t-23.500674\t0.370000\t0.075000\n\t\n15:20:53.4\tlog_raw\tgps_raw\t#DUALANTENNAHEADINGA,USB3,0,47.0,FINESTEERING,2107,282071.400,02008000,d426,15824;SOL_COMPUTED,NARROW_FLOAT,-1.000000000,165.423980713,-15.767028809,0.0,239.021484375,180.000000000,\"631T\",20,7,7,7,04,00,20,03*cfd53cf7\n\tsystem status\tnormal 2 28.000000 0 0\trobot status\t245.941408\t97.044518\t8.474600\t0.240054\t0.979310\t-23.961822\t0.345000\t0.044000\n\t\n15:20:53.9\tlog_raw\tgps_raw\t#DUALANTENNAHEADINGA,USB3,0,47.0,FINESTEERING,2107,282071.900,02008000,d426,15824;SOL_COMPUTED,NARROW_FLOAT,-1.000000000,165.887359619,-16.480316162,0.0,236.674011230,180.000000000,\"631T\",20,7,7,7,04,00,20,03*dd935a36\n\tsystem status\tnormal 2 28.000000 0 0\trobot status\t246.068492\t96.976592\t8.478100\t0.102486\t0.776770\t-24.544194\t0.342000\t0.040000\n\t\n15:20:54.4\tlog_raw\tgps_raw\t#DUALANTENNAHEADINGA,USB3,0,49.5,FINESTEERING,2107,282072.400,02008000,d426,15824;SOL_COMPUTED,NARROW_FLOAT,-1.000000000,175.843307495,41.730823517,0.0,200.143447876,180.000000000,\"631T\",21,7,7,7,04,00,20,03*fbe9d2f7\n\tsystem status\tnormal 2 28.000000 0 0\trobot status\t246.193820\t96.907963\t8.480900\t0.108534\t0.662227\t-25.260349\t0.232000\t-0.115000\n\t\n15:20:54.9\tlog_raw\tgps_raw\t#DUALANTENNAHEADINGA,USB3,0,49.5,FINESTEERING,2107,282072.900,02008000,d426,15824;SOL_COMPUTED,NARROW_FLOAT,-1.000000000,175.657180786,43.295608521,0.0,201.745788574,180.000000000,\"631T\",21,7,7,7,04,00,20,03*de4c8f7d\n\tsystem status\tnormal 2 28.000000 0 0\trobot status\t246.318857\t96.836488\t8.482600\t0.209753\t0.542815\t-25.981699\t0.309000\t0.006000\n\t\n15:20:55.4\tlog_raw\tgps_raw\t#DUALANTENNAHEADINGA,USB3,0,50.0,FINESTEERING,2107,282073.400,02008000,d426,15824;SOL_COMPUTED,NARROW_FLOAT,-1.000000000,88.259048462,72.880012512,0.0,360.000000000,91.084091187,\"631T\",19,7,7,7,04,00,20,03*7543b6a9\n\tsystem status\tnormal 2 28.000000 0 0\trobot status\t246.440976\t96.766535\t8.486100\t0.131852\t0.358068\t-26.629710\t0.285000\t-0.029000\n\t\n15:20:55.9\tlog_raw\tgps_raw\t\tsystem status\tnormal 2 28.000000 0 0\trobot status\t246.561048\t96.695943\t8.488400\t0.048518\t0.452481\t-27.261197\t0.283000\t-0.037000\n\t\n15:20:56.4\tlog_raw\tgps_raw\t#DUALANTENNAHEADINGA,USB3,0,48.5,FINESTEERING,2107,282074.400,02000000,d426,15824;SOL_COMPUTED,NARROW_FLOAT,-1.000000000,187.625686646,-11.833007813,0.0,215.399688721,180.000000000,\"631T\",19,7,7,7,04,00,20,03*14c71104\n\tsystem status\tnormal 2 28.000000 0 0\trobot status\t246.682726\t96.622612\t8.489900\t0.064089\t0.351975\t-27.864520\t0.301000\t0.009000\n\t\n15:20:56.9\tlog_raw\tgps_raw\t\tsystem status\tnormal 2 28.000000 0 0\trobot status\t246.803458\t96.549781\t8.491400\t-0.002376\t0.199417\t-28.322294\t0.352000\t0.070000\n\t\n
